vi "Read Options Selection (SubVI).vi"() -> (3 "Options Selection":i32[](array[numeric]))   [LabVIEW 2020]
uses:
  <vilib>/Utility/config.llb/Read Key (I32).vi
  <vilib>/Utility/config.llb/Write Key (I32).vi
  <vilib>/Utility/config.llb/NI_LVConfig.lvlib
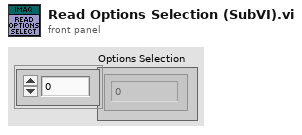
[diagram p1: front panel]
types:
  T1 = typedef "NI_LVConfig.lvlib/Config Data RefNum.ctl" = refnum<k1>
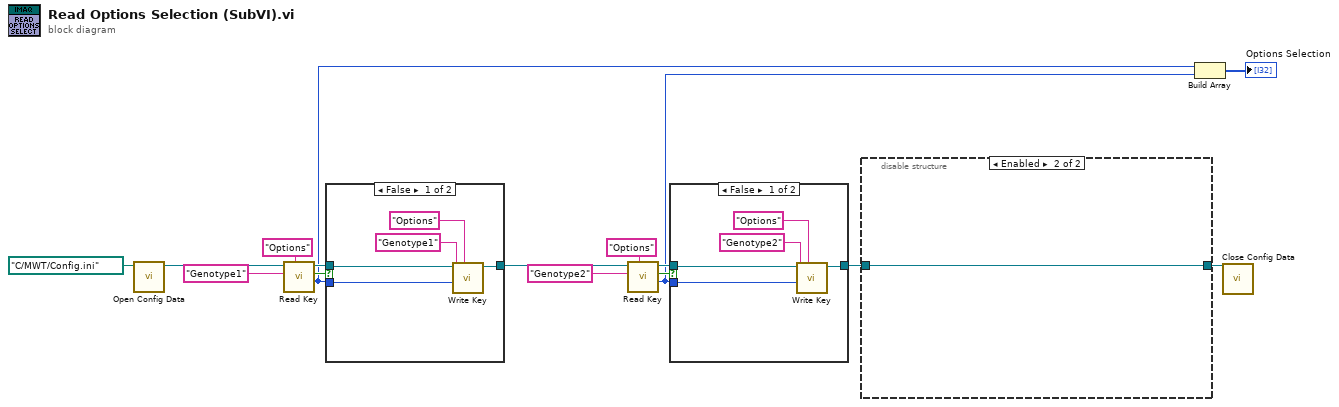
[diagram p0: block diagram]
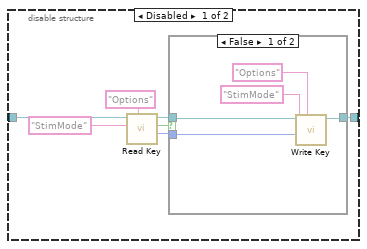
[diagram p2: hidden frame]
diagram:
  n1 = call <vilib>:"Open Config Data.vi"("configuration file path"=path "C:/MWT/Config.ini") -> ("refnum"=w14:T1)  [unwired: 8 in, 2 out]
  n2 = call-poly <vilib>:"Read Key.vi"("section"="Options", "key"="Genotype1" ("section"), "refnum"=w14) -> ("value"=w3:i32, "found?"=w12:bool, "refnum out"=w11:T1)  [unwired: 5 in, 1 out]
  n3 = case shown="False" w12 {
    tunnel: w11 -> [w19 w22]
    tunnel: [w18 w22] -> w6
    tunnel: w3 -> [w17 _]
    frame False {
      n4 = call-poly <vilib>:"Write Key.vi"("section"="Options", "value"=w17, "key"="Genotype1" ("section"), "refnum"=w19) -> ("refnum out"=w18:T1)  [unwired: 5 in, 2 out]
    }
    frame True {
    }
  }
  n5 = call-poly <vilib>:"Read Key.vi"("section"="Options", "key"="Genotype2" ("section"), "refnum"=w6) -> ("value"=w2:i32, "found?"=w9:bool, "refnum out"=w10:T1)  [unwired: 5 in, 1 out]
  n6 = case shown="False" w9 {
    tunnel: w10 -> [w25 w28]
    tunnel: [w24 w28] -> w5
    tunnel: w2 -> [w23 _]
    frame False {
      n7 = call-poly <vilib>:"Write Key.vi"("section"="Options", "value"=w23, "key"="Genotype2" ("section"), "refnum"=w25) -> ("refnum out"=w24:T1)  [unwired: 5 in, 2 out]
    }
    frame True {
    }
  }
  n8 = disable-structure shown="Enabled" {
    disable-tunnel: w5 -> [w31 w42]
    disable-tunnel: [w30 w42] -> w4
    frame Disabled {
      n9 = call-poly <vilib>:"Read Key.vi"("section"="Options", "key"="StimMode" ("section"), "refnum"=w31) -> ("value"=w29:i32, "found?"=w33:bool, "refnum out"=w32:T1)  [unwired: 5 in, 1 out]
      n10 = case shown="False" w33 {
        tunnel: w32 -> [w38 w41]
        tunnel: [w37 w41] -> w30
        tunnel: w29 -> [w36 _]
        frame False {
          n11 = call-poly <vilib>:"Write Key.vi"("section"="Options", "value"=w36, "key"="StimMode" ("section"), "refnum"=w38) -> ("refnum out"=w37:T1)  [unwired: 5 in, 2 out]
        }
        frame True {
        }
      }
    }
    frame Enabled {
    }
  }
  n12 = Build Array(w3, w2) -> (→"Options Selection":i32[])
  n13 = call <vilib>:"Close Config Data.vi"("refnum"=w4) -> ()  [unwired: 9 in, 2 out]
